vi "Stop InterComm.vi"(8 "error in (no error)":errorcluster, 11 "Messenger in":refnum<class "Messenger.lvclass">) -> (0 "error out":errorcluster, 3 "Messenger out":refnum<class "Messenger.lvclass">)   [LabVIEW 2018, in "Messenger.lvclass"]
uses:
  Messenger.lvclass
  Messenger.lvclass/Messenger.ctl
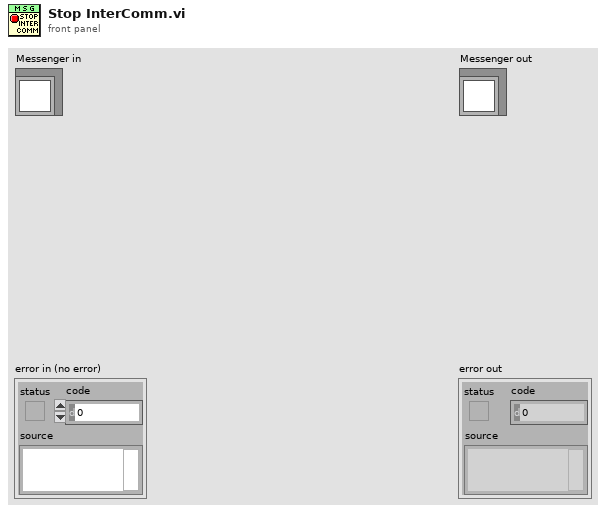
[diagram p1: front panel]
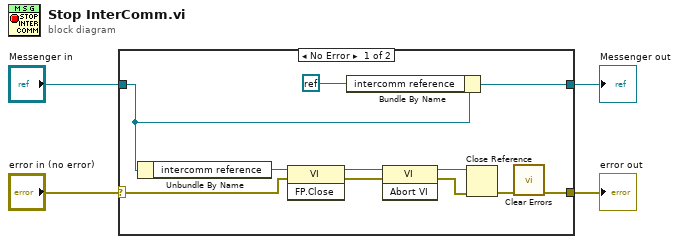
[diagram p0: block diagram]
diagram:
  n1 = case shown="No Error" "error in (no error)" {
    selector: "error in (no error)" -> [w11 w16]
    tunnel: [w8 w16] -> w3
    tunnel: [w6 w17] -> w1
    tunnel: "Messenger in" -> [w7 w17]
    frame No Error {
      n2 = Unbundle By Name(w7) -> ("intercomm reference"=w12:refnum<vi>)
      n3 = invoke class="VI" method="FP.Close"(reference=w12, error in=w11) -> (reference out=w15:refnum<vi>, error out=w13:errorcluster)  [unwired: 1 in, 1 out]
      n4 = Bundle By Name(cluster=w7, "intercomm reference"=refnum<k0> refnum) -> (w6:refnum<class "Messenger.lvclass">)
      n5 = invoke class="VI" method="Abort VI"(reference=w15, error in=w13) -> (reference out=w14:refnum<vi>, error out=w10:errorcluster)  [unwired: 1 in, 1 out]
      n6 = Close Reference(reference=w14, error in (no error)=w10) -> (error out=w9:errorcluster)
      n7 = call <vilib>:"Clear Errors.vi"("error in (no error)"=w9) -> ("error out"=w8:errorcluster)  [unwired: 5 in, 1 out]
    }
    frame Error {
    }
  }
  "error out" <- w3
  "Messenger out" <- w1
